vi "prepare server.vi"(8 "error in":errorcluster, 9 "max allowed":i32, 10 "connection string":string, 11 "connection server in":refnum<class "connection server.lvclass">) -> (0 "error out":errorcluster, 3 "connection server out":refnum<class "connection server.lvclass">)   [LabVIEW 2015, in "connection server.lvclass"]
uses:
  connection server.lvclass
  connection server.lvclass/connection server.ctl
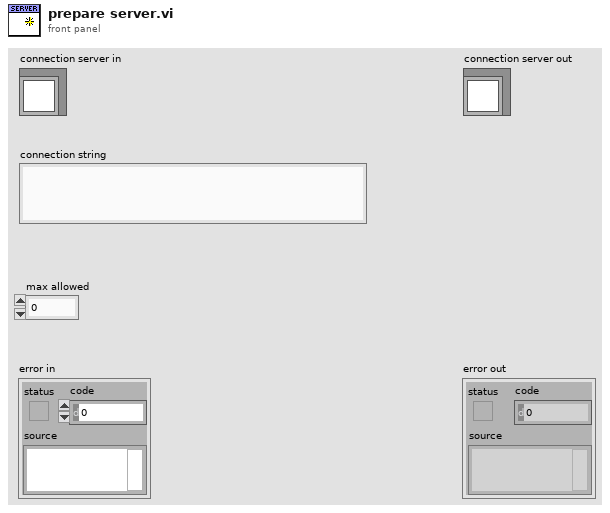
[diagram p1: front panel]
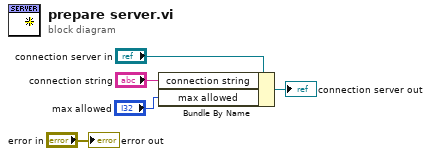
[diagram p0: block diagram]
diagram:
  n1 = Bundle By Name(cluster="connection server in", "connection string"="connection string", "max allowed"="max allowed") -> (→"connection server out":refnum<class "connection server.lvclass">)
  "error out" <- "error in"
